vi "HFRR ADV v02.vi"() -> ()   [LabVIEW 2023] (continued)
            n1522 = Concatenate Strings("(" ("string"), w1758, ")  Deg C ," ("string")) -> (w1757:string)
            n1523 = Concatenate Strings("(" ("string"), w1754, " ) % RH," ("string")) -> (w1753:string)
            n1524 = Concatenate Strings("(" ("string"), w1750, ")  Deg C ," ("string")) -> (w1749:string)
            n1525 = Concatenate Strings("(" ("string"), w1747, ")  Microns," ("string")) -> (w1746:string)
            n1526 = local read "REMARKS"() -> (w1767:string)
            "REMARKS 2" <- w1767
            n1527 = Concatenate Strings(w1767, w1732, " Humidity before test= " ("Substring"), w1762, w1732, " Temperature before test = " ("Substring"), w1757, w1732, " Humidity after test= " ("Substring"), w1753, w1732, "Temperature after test = " ("Substring"), w1749, w1732, "MSD = " ("Substring"), w1746, w1732, "  AVP = " ("Substring"), w1733, w1732, "  HCF                     =( " ("Substring"), w1739, w1732, " WS1.4                  = " ("Substring"), w1735, w1732) -> (w1731:string)
            "data" <- w1731
            n1528 = call <vilib>:"Write Characters To File.vi"("append to file? (new file:F)"=FALSE, "character string"=w1731, "file path (dialog if empty)"=w1784) -> ()  [unwired: 2 in, 1 out]
            n1529 = Match Pattern(string=w1731, regular expression="!") -> (after substring=→"export":string)  [unwired: 1 in, 3 out]
          }
        }
        n1530 = local read "Temperature before test"() -> (w1700:dbl)
        n1531 = local read "Humidity before test"() -> (w1702:dbl)
        n1532 = local read "Temperature after test"() -> (w1716:dbl)
        n1533 = Add(x=231.864, y=w1700) -> (x+y=w1697:dbl)
        n1534 = Add(x=231.864, y=w1716) -> (x+y=w1713:dbl)
        n1535 = local read "Humidity after test"() -> (w1718:dbl)
        n1536 = Divide(x=1705.984, y=w1697) -> (x/y=w1698:dbl)
        n1537 = Divide(x=1705.984, y=w1713) -> (x/y=w1714:dbl)
        n1538 = Subtract(x=8.017352 ("y"), y=w1698) -> (x-y=w1727:dbl)
        n1539 = expression code="10**y"(w1727) -> (w1704:dbl)
        n1540 = Subtract(x=8.017352 ("y"), y=w1714) -> (x-y=w1721:dbl)
        n1541 = expression code="10**y"(w1721) -> (w1720:dbl)
        n1542 = Multiply(x=w1702, y=w1704) -> (x*y=w1703:dbl)
        n1543 = Multiply(x=w1718, y=w1720) -> (x*y=w1719:dbl)
        n1544 = Divide(x=w1703, y=750.0) -> (x/y=w1722:dbl)
        n1545 = Divide(x=w1719, y=750.0) -> (x/y=w1723:dbl)
        n1546 = Add(x=w1722, y=w1723) -> (x+y=w1724:dbl)
        n1547 = Divide(x=w1724, y=2.0) -> (x/y=w1726:dbl)
        n1548 = local write "AVP"(w1726) -> ()
        n1549 = local read "HCF"() -> (w1709:dbl)
        n1550 = Subtract(x=1.4, y=w1726) -> (x-y=w1707:dbl)
        n1551 = local read "MWSD"() -> (w1705:dbl)
        n1552 = Multiply(x=w1707, y=w1709) -> (x*y=w1708:dbl)
        n1553 = Add(x=w1708, y=w1705) -> (x+y=→"WS1.4":dbl)
      }
    }
    n1554 = case shown="True" "Prog Uno" {
      frame False {
      }
      frame True {
        n1555 = stacked-sequence {
          frame #0 {
            n1556 = Delete(path (use dialog)=path "C:/LAB-IQ-NXT/UNOCOMPILE.bat" ("working directory")) -> ()  [unwired: 4 in, 3 out]
          }
          frame #1 {
            n1557 = local read "Com Port 1"() -> (w1297:refnum<visa-resource-name>)
            n1558 = Concatenate Strings("cmd.exe /c \"mode " ("command line"), w1297, ":1200,n,8,1\"\n" ("command line")) -> (w1302:string)
            n1559 = Concatenate Strings(w1302, "CD\\\nCD WinDucom\navrdude -C avrdude.conf -v -patmega328p -carduino -P" ("command line"), w1297, " -b115200 -D -Uflash:w:UNO_V20.hex:i\n" ("command line"), "\r") -> (w1304:string)
            "STR" <- w1304
            n1560 = call <vilib>:"Write Characters To File.vi"("append to file? (new file:F)"=FALSE, "character string"=w1304, "file path (dialog if empty)"=path "C:/LAB-IQ-NXT/UNOCOMPILE.bat" ("working directory")) -> ()  [unwired: 2 in, 1 out]
          }
          frame #2 {
            n1561 = case shown="True" "Case Constant\n(See Context Help) 10" {
              frame False {
              }
              frame True {
                w1310 = "cmd.exe  /c \"C:\\LAB-IQ-NXT\\UNOCOMPILE.bat\"" ("string")
                n1562 = call <vilib>:"System Exec.vi"("expected output size  (4096)"=u32 65535, "run minimized? (F)"=FALSE, "wait until completion? (T)"=TRUE ("run minimized? (F)"), "working directory"=path "C:/LAB-IQ-NXT", "standard input"=w1310, "command line"=w1310) -> ("error out"=w1309:errorcluster, "standard output"=→"String 42":string)  [unwired: 2 in, 2 out]
                "error out 3" <- w1309
                n1563 = flat-sequence {
                  tunnel: w1309 -> [_]
                  frame #0 {
                  }
                }
              }
            }
            n1564 = local write "Prog Uno"(FALSE ("run minimized? (F)")) -> ()
          }
        }
      }
    }
    n1565 = case shown="True" "Prog Due" {
      frame False {
      }
      frame True {
        n1566 = stacked-sequence {
          frame #0 {
            n1567 = Delete(path (use dialog)=path "C:/LAB-IQ-NXT/DUECOMPILE.bat" ("working directory")) -> ()  [unwired: 4 in, 3 out]
          }
          frame #1 {
            n1568 = case shown="True" "Case Constant\n(See Context Help) 11" {
              frame False {
              }
              frame True {
                n1569 = local read "visa due"() -> (w1278:string)
                n1570 = Concatenate Strings("cmd.exe /c \"mode " ("command line"), w1278, ":1200,n,8,1\"\n" ("command line")) -> (w1283:string)
                n1571 = Concatenate Strings(w1283, "CD\\\nCD WinDucom\nTIMEOUT 1\n bossac.exe -i -d --port=" ("command line"), w1278, " -U false -e -w -v -b DUE.bin -R\n" ("command line"), "\r") -> (w1285:string)
                "concatenated string 2" <- w1285
                n1572 = call <vilib>:"Write Characters To File.vi"("append to file? (new file:F)"=FALSE, "character string"=w1285, "file path (dialog if empty)"=path "C:/LAB-IQ-NXT/DUECOMPILE.bat" ("working directory")) -> ()  [unwired: 2 in, 1 out]
              }
            }
          }
          frame #2 {
            # "C:\\LAB-IQ-NXT\\DUECOMPILE.bat"
            n1573 = case shown="True" "Case Constant\n(See Context Help) 12" {
              frame False {
              }
              frame True {
                w1291 = "cmd.exe  /c \"C:\\LAB-IQ-NXT\\DUECOMPILE.bat\"" ("string")
                n1574 = call <vilib>:"System Exec.vi"("expected output size  (4096)"=u32 65535, "run minimized? (F)"=FALSE, "wait until completion? (T)"=TRUE ("run minimized? (F)"), "working directory"=path "C:/LAB-IQ-NXT", "standard input"=w1291, "command line"=w1291) -> ("error out"=w1290:errorcluster, "standard output"=→"String 44":string)  [unwired: 2 in, 2 out]
                "error out 4" <- w1290
                n1575 = flat-sequence {
                  tunnel: w1290 -> [_]
                  frame #0 {
                  }
                }
              }
            }
            n1576 = local write "Prog Due"(FALSE ("Prog Due")) -> ()
          }
        }
      }
    }
    n1577 = flat-sequence {
      frame #0 {
        n1578 = local read "x = y?"() -> (w1320:bool)
        n1579 = And(x="EDIT", y=w1320) -> (x .and. y?=w1318:bool)
        n1580 = case shown="True" "SAVE" {
          frame False {
          }
          frame True {
            n1581 = stacked-sequence {
              seq-local: [w1521 _ _] -> [_ w1677 _]
              frame #0 {
                (unwired) i16 5 ("precision (6)")
                # "[CH1]    - FF\n[CH2]   - TEMPERATURE\n[CH3]    - Humidity\n[CH4]    - AIR TEMP\n[CH5]\\- Visa Uno\n[CH6] \\- Visa Due\n[CH7]  \\- file path\n[CH8]   - Displacement Gain\n[CHA]   - Stroke Gain\n[CHB]   - Stroke PID Gain\n[CHC]   -Language Selection\n[CHD]   -Power +\n[CHE]   -Power_\n[CHF]   -Heater\n[CHG]   -Humidity Wet\n[CHH]   -Humidity Dry\n[CHI]   -Integral Time"
                n1582 = local read "Com Port 1"() -> (w1512:refnum<visa-resource-name>)
                n1583 = local read "AIR TEMPERATURE :"() -> (w1508:dbl)
                n1584 = local read "DISPLACEMENT :"() -> (w1506:dbl)
                n1585 = local read "HUMIDITY:"() -> (w1507:dbl)
                n1586 = local read "Com Port 2"() -> (w1511:refnum<visa-resource-name>)
                n1587 = local read "TEMPERATURE :"() -> (w1509:dbl)
                n1588 = local read "Stroke PID Gains"() -> (w1572:T5)
                n1589 = local read "FRIC. FORCE :"() -> (w1510:dbl)
                n1590 = local read "STROKE GAIN :"() -> (w1505:dbl)
                n1591 = Unbundle By Name(w1572) -> ("Proportional Gain (Kc)"=w1571:dbl, "Integral Time (Ti, min)"=w1513:dbl)
                n1592 = local read "CH-HUMIDITY DRY"() -> (w1524:u16)
                n1593 = Path To String(path="File Path") -> (string=w1594:string)
                n1594 = local read "Language Selection"() -> (w1569:enum16{"English", "Russian"})
                n1595 = local read "CH-POWER +"() -> (w1536:u16)
                n1596 = local read "CH-HUMIDITY WET"() -> (w1527:u16)
                n1597 = Number To Fractional String(number=w1507, width (-)=i16 10 ("precision (6)"), precision (6)=i16 5) -> (F-format string=w1619:string)  [unwired: 1 in]
                n1598 = Concatenate Strings(w1594, "\\" ("string")) -> (w1593:string)
                n1599 = local read "CH-POWER -"() -> (w1533:u16)
                n1600 = Number To Fractional String(number=w1509, width (-)=i16 10 ("precision (6)"), precision (6)=i16 5) -> (F-format string=w1625:string)  [unwired: 1 in]
                n1601 = Number To Fractional String(number=w1508, width (-)=i16 10 ("precision (6)"), precision (6)=i16 5) -> (F-format string=w1613:string)  [unwired: 1 in]
                n1602 = Number To Fractional String(number=w1506, width (-)=i16 10 ("precision (6)"), precision (6)=i16 5) -> (F-format string=w1586:string)  [unwired: 1 in]
                n1603 = local read "CH-HEATER"() -> (w1530:u16)
                n1604 = Number To Fractional String(number=w1505, width (-)=i16 10 ("precision (6)"), precision (6)=i16 5) -> (F-format string=w1585:string)  [unwired: 1 in]
                n1605 = Number To Fractional String(number=w1510, width (-)=i16 10 ("precision (6)"), precision (6)=i16 5) -> (F-format string=w1626:string)  [unwired: 1 in]
                n1606 = Number To Fractional String(number=w1571, width (-)=i16 10 ("precision (6)"), precision (6)=i16 5) -> (F-format string=w1573:string)  [unwired: 1 in]
                n1607 = Number To Fractional String(number=w1569, width (-)=i16 10 ("precision (6)"), precision (6)=i16 5) -> (F-format string=w1565:string)  [unwired: 1 in]
                n1608 = Number To Fractional String(number=w1536, width (-)=i16 10 ("precision (6)"), precision (6)=i16 5) -> (F-format string=w1559:string)  [unwired: 1 in]
                n1609 = Number To Fractional String(number=w1533, width (-)=i16 10 ("precision (6)"), precision (6)=i16 5) -> (F-format string=w1556:string)  [unwired: 1 in]
                n1610 = Number To Fractional String(number=w1530, width (-)=i16 10 ("precision (6)"), precision (6)=i16 5) -> (F-format string=w1551:string)  [unwired: 1 in]
                n1611 = Number To Fractional String(number=w1527, width (-)=i16 10 ("precision (6)"), precision (6)=i16 5) -> (F-format string=w1548:string)  [unwired: 1 in]
                n1612 = Number To Fractional String(number=w1524, width (-)=i16 10 ("precision (6)"), precision (6)=i16 5) -> (F-format string=w1543:string)  [unwired: 1 in]
                n1613 = Concatenate Strings("[CH1]" ("string"), w1626, " - FF" ("string"), "\r") -> (w1624:string)
                n1614 = Concatenate Strings("[CH3]" ("string"), w1619, " - Humidity" ("string"), "\r") -> (w1616:string)
                n1615 = Concatenate Strings("[CH7]" ("string"), w1593, "- file path" ("string"), "\r") -> (w1596:string)
                n1616 = Number To Fractional String(number=w1513, width (-)=i16 10 ("precision (6)"), precision (6)=i16 5) -> (F-format string=w1517:string)  [unwired: 1 in]
                n1617 = Concatenate Strings("[CH6]" ("string"), w1511, "- Visa Due" ("string"), "\r") -> (w1597:string)
                n1618 = Concatenate Strings("[CH8]" ("string"), w1586, "- Displacement Gain" ("string"), "\r") -> (w1589:string)
                n1619 = Concatenate Strings("[CHA]" ("string"), w1585, "- Stroke Gain" ("string"), "\r") -> (w1579:string)
                n1620 = Concatenate Strings("[CH5]" ("string"), w1512, "- Visa Uno" ("string"), "\r") -> (w1602:string)
                n1621 = Concatenate Strings("[CH4]" ("string"), w1613, " - AIR TEMP" ("string"), "\r") -> (w1609:string)
                n1622 = Concatenate Strings("[CH2]" ("string"), w1625, " - TEMPERATURE" ("string"), "\r") -> (w1623:string)
                n1623 = Concatenate Strings("[CHC]" ("string"), w1565, "-Language Selection" ("string"), "\r") -> (w1562:string)
                n1624 = Concatenate Strings("[CHD]" ("string"), w1559, "-Power +" ("string"), "\r") -> (w1541:string)
                n1625 = Concatenate Strings("[CHE]" ("string"), w1556, "-Power_" ("string"), "\r") -> (w1540:string)
                n1626 = Concatenate Strings("[CHF]" ("string"), w1551, "-Heater" ("string"), "\r") -> (w1539:string)
                n1627 = Concatenate Strings("[CHB]" ("string"), w1573, "- Stroke PID Gain" ("string"), "\r") -> (w1570:string)
                n1628 = Concatenate Strings("[CHG]" ("string"), w1548, "-Humidity Wet" ("string"), "\r") -> (w1538:string)
                n1629 = Concatenate Strings("[CHH]" ("string"), w1543, "-Humidity Dry" ("string"), "\r") -> (w1537:string)
                n1630 = Concatenate Strings("[CHI]" ("string"), w1517, "-Integral Time " ("string"), "\r") -> (w1514:string)
                n1631 = Concatenate Strings(w1624, w1623, w1616, w1609, w1602, w1597, w1596, w1589, w1579, w1570, w1562, w1541, w1540, w1539, w1538, w1537, w1514) -> (w1521:string)
                "gain" <- w1521
              }
              frame #1 {
                n1632 = local read "AIR TEMP INTERCEPT:"() -> (w1638:dbl)
                n1633 = local read "TEMP INTERCEPT:"() -> (w1637:dbl)
                n1634 = local read "Com Port 3"() -> (w1647:refnum<visa-resource-name>)
                n1635 = local read "LvdtOff"() -> (w1640:dbl)
                n1636 = Number To Fractional String(number=w1637, width (-)=i16 10 ("precision (6)"), precision (6)=i16 5) -> (F-format string=w1665:string)  [unwired: 1 in]
                n1637 = Number To Fractional String(number=w1638, width (-)=i16 10 ("precision (6)"), precision (6)=i16 5) -> (F-format string=w1672:string)  [unwired: 1 in]
                n1638 = Number To Fractional String(number=w1640, width (-)=i16 10 ("precision (6)"), precision (6)=i16 5) -> (F-format string=w1644:string)  [unwired: 1 in]
                n1639 = Concatenate Strings("[CHK]" ("string"), w1665, "-TEMP INTERCEPT" ("string"), "\r") -> (w1661:string)
                n1640 = Concatenate Strings("[CHJ]" ("string"), w1672, "-AIR TEMP INTERCEPT" ("string"), "\r") -> (w1662:string)
                n1641 = Concatenate Strings("[SNO]" ("string"), "S.NO", "-" ("string"), "\r") -> (w1657:string)
                n1642 = Concatenate Strings("[CHL]" ("string"), w1647, "- Visa humid" ("string"), "\r") -> (w1650:string)
                n1643 = Concatenate Strings("[CHI]" ("string"), w1644, "-LVDT Position Offset" ("string"), "\r") -> (w1639:string)
                n1644 = Concatenate Strings(w1677, w1662, w1661, w1657, w1650, w1639) -> (w1676:string)
                n1645 = local read "Gain path"() -> (w1655:string)
                n1646 = Concatenate Strings(w1655, "\\calibrate std ED hfrr.dcf") -> ()  [unwired: 1 out]
                n1647 = String To Path(string="C:\\LAB-IQ-NXT\\calibrate WO 2464.dcf") -> (path=w1648:path)
                n1648 = call <vilib>:"Write Characters To File.vi"("append to file? (new file:F)"=FALSE, "character string"=w1676, "file path (dialog if empty)"=w1648) -> ()  [unwired: 2 in, 1 out]
              }
              frame #2 {
                n1649 = local write "Lan flag"(0.0 ("Lan flag")) -> ()
                n1650 = local write "Re-Initialise"(TRUE ("Re-Initialise")) -> ()
                n1651 = local write "conststatus"(0.0 ("rpm value : 2")) -> ()
                n1652 = local write "SAVE"(FALSE ("OK Button 14")) -> ()
              }
            }
          }
        }
        n1653 = case shown="False" w1318 {
          tunnel: [u8 2 ("Disabled") u8 0 ("Disabled")] -> w1317
          tunnel: [w1682 TRUE ("Visible")] -> w1316
          frame False {
            w1682 = FALSE ("Visible")
            n1654 = local write "EDIT 2"(w1682) -> ()
          }
          frame True {
          }
        }
        n1655 = property on="Tab Control" class="TabCtl (strict)"("Visible"=w1316) -> ()  [unwired: 2 in, 2 out]
        n1656 = property on="EDIT 2" class="Bool (strict)"("Visible"=w1316) -> ()  [unwired: 2 in, 2 out]
        n1657 = property on="TEMPERATURE :" class="DigNum (strict)"("Disabled"=w1317) -> ()  [unwired: 2 in, 2 out]
        n1658 = property on="SAVE" class="Bool (strict)"("Visible"=w1316) -> ()  [unwired: 2 in, 2 out]
        n1659 = property on="AIR TEMPERATURE :" class="DigNum (strict)"("Disabled"=w1317) -> ()  [unwired: 2 in, 2 out]
        n1660 = property on="SPEED OUT:" class="DigNum (strict)"("Disabled"=w1317) -> ()  [unwired: 2 in, 2 out]
        n1661 = property on="HUMIDITY:" class="DigNum (strict)"("Disabled"=w1317) -> ()  [unwired: 2 in, 2 out]
        n1662 = property on="FRIC. FORCE :" class="DigNum (strict)"("Disabled"=w1317) -> ()  [unwired: 2 in, 2 out]
        n1663 = property on="Tab Control 7" class="TabCtl (strict)"("Disabled"=w1317) -> ()  [unwired: 2 in, 2 out]
        n1664 = property on="Language Selection" class="Enum (strict)"("Visible"=w1316) -> ()  [unwired: 2 in, 2 out]
        n1665 = property on="File Path" class="Path"("Disabled"=w1317) -> ()  [unwired: 2 in, 2 out]
        n1666 = property on="TEMP INTERCEPT:" class="DigNum (strict)"("Disabled"=w1317) -> ()  [unwired: 2 in, 2 out]
        n1667 = property on="visa due" class="CmbBox"("Disabled"=w1317) -> ()  [unwired: 2 in, 2 out]
        n1668 = property on="AIR TEMP INTERCEPT:" class="DigNum (strict)"("Disabled"=w1317) -> ()  [unwired: 2 in, 2 out]
        n1669 = property on="CH-HUMIDITY DRY" class="DigNum (strict)"("Disabled"=w1317) -> ()  [unwired: 2 in, 2 out]
        n1670 = property on="CH-HUMIDITY WET" class="DigNum (strict)"("Disabled"=w1317) -> ()  [unwired: 2 in, 2 out]
        n1671 = property on="CH-POWER -" class="DigNum (strict)"("Disabled"=w1317) -> ()  [unwired: 2 in, 2 out]
        n1672 = property on="CH-HEATER" class="DigNum (strict)"("Disabled"=w1317) -> ()  [unwired: 2 in, 2 out]
        n1673 = property on="CH-POWER +" class="DigNum (strict)"("Disabled"=w1317) -> ()  [unwired: 2 in, 2 out]
        n1674 = property on="SrvM CP" class="Bool (strict)"("Disabled"=w1317) -> ()  [unwired: 2 in, 2 out]
        n1675 = property on="Stroke PID Gains" class="Clust (strict)"("Disabled"=w1317) -> ()  [unwired: 2 in, 2 out]
        n1676 = property on="STROKE GAIN :" class="DigNum (strict)"("Disabled"=w1317) -> ()  [unwired: 2 in, 2 out]
        n1677 = property on="LvdtOff" class="DigNum (strict)"("Disabled"=w1317) -> ()  [unwired: 2 in, 2 out]
        n1678 = property on="DISPLACEMENT :" class="DigNum (strict)"("Disabled"=w1317) -> ()  [unwired: 2 in, 2 out]
        n1679 = property on="Port 2 Error" class="Clust (strict)"("Visible"="EDIT") -> ()  [unwired: 2 in, 2 out]
        n1680 = property on="Port 1 Error" class="Clust (strict)"("Visible"="EDIT") -> ()  [unwired: 2 in, 2 out]
        n1681 = stacked-sequence {
          frame #0 {
            n1682 = local read "EDIT"() -> (w1368:bool)
            n1683 = case shown="False" w1368 {
              tunnel: [u8 2 ("Disabled") u8 0 ("Disabled")] -> _
              frame False {
                w1370 = FALSE
                n1684 = local write "Password"("") -> ()
                n1685 = property on="ENTER THE NEW PASSWORD" class="Str"("Visible"=w1370) -> ()  [unwired: 2 in, 2 out]
                n1686 = property on="ENTER CURRENT PASSWORD" class="Str"("Visible"=w1370) -> ()  [unwired: 2 in, 2 out]
                n1687 = property on="SrvM CP" class="Bool (strict)"("Visible"=w1370) -> ()  [unwired: 2 in, 2 out]
                n1688 = property on="Password" class="Str"("Visible"=w1370) -> ()  [unwired: 2 in, 2 out]
                n1689 = local write "x = y?"(w1370) -> ()
                n1690 = local write "SrvM CP"(w1370) -> ()
                n1691 = property on="message" class="Str"("Visible"=w1370) -> ()  [unwired: 2 in, 2 out]
              }
              frame True {
                w1373 = TRUE
                n1692 = property on="SrvM CP" class="Bool (strict)"("Visible"=w1373) -> ()  [unwired: 2 in, 2 out]
                n1693 = property on="Password" class="Str"("Visible"=w1373) -> ()  [unwired: 2 in, 2 out]
              }
            }
            "dipl pwd" <- "@143$\n" ("dipl pwd")
          }
          frame #1 {
            # "Gain password"
            n1694 = String To Byte Array(string="ENTER CURRENT PASSWORD") -> (unsigned byte array=w1378:u8[])
            n1695 = Search 1D Array(1D array=w1378, element=u8 10) -> (index of element=w1381:i32)  [unwired: 1 in]
            n1696 = Index Array(array=w1378, index=w1381) -> (element=w1377:u8)
            n1697 = Equal?(x=w1377, y=10) -> (x = y?=w1375:bool)
            n1698 = case shown="True" w1375 {
              frame False {
                n1699 = property on="ENTER THE NEW PASSWORD" class="Str"("Visible"=FALSE) -> ()  [unwired: 2 in, 2 out]
              }
              frame True {
                # "password"
                # "change password logic"
                n1700 = local read "dipl pwd"() -> (w1388:string)
                n1701 = local read "ENTER CURRENT PASSWORD"() -> (w1394:string)
                n1702 = String To Byte Array(string=w1394) -> (unsigned byte array=w1396:u8[])
                n1703 = Array Size(array=w1396) -> (size(s)=w1393:i32)
                n1704 = String To Byte Array(string=w1388) -> (unsigned byte array=w1389:u8[])
                n1705 = Array Size(array=w1389) -> (size(s)=w1391:i32)
                n1706 = for {
                  N: w1393 -> [_]
                  tunnel: w1396 -> [w1420]
                  tunnel: [w1418] -> w1397 mode=indexing
                  tunnel: w1393 -> [w1412]
                  i -> [w1413]
                  n1707 = Decrement(x=w1412) -> (x-1=w1410:i32)
                  n1708 = Index Array(array=w1420, index=w1413) -> (element=w1414:u8)
                  n1709 = Equal?(x=w1413, y=w1410) -> (x = y?=w1411:bool)
                  n1710 = Number To Decimal String(number=w1414) -> (decimal integer string=w1419:string)  [unwired: 1 in]
                  n1711 = Select(t="", s=w1411, f="\r") -> (s? t:f=w1416:string)
                  n1712 = Concatenate Strings(w1419, w1416) -> (w1418:string)
                }
                n1713 = for {
                  N: w1391 -> [_]
                  tunnel: w1389 -> [w1408]
                  tunnel: [w1406] -> w1390 mode=indexing
                  tunnel: w1391 -> [w1403]
                  i -> [w1404]
                  n1714 = Decrement(x=w1403) -> (x-1=w1402:i32)
                  n1715 = Index Array(array=w1408, index=w1404) -> (element=w1407:u8)
                  n1716 = Equal?(x=w1404, y=w1402) -> (x = y?=w1401:bool)
                  n1717 = Number To Decimal String(number=w1407) -> (decimal integer string=w1405:string)  [unwired: 1 in]
                  n1718 = Select(t="", s=w1401, f="\r") -> (s? t:f=w1398:string)
                  n1719 = Concatenate Strings(w1405, w1398) -> (w1406:string)
                }
                n1720 = local read "string"() -> (w1395:string)
                n1721 = Concatenate Strings(w1397) -> (w1385:string)
                n1722 = Concatenate Strings(w1390) -> (w1384:string)
                n1723 = Concatenate Strings(w1395) -> (w1392:string)
                n1724 = Equal?(x=w1385, y=w1384) -> (x = y?=w1383:bool)
                n1725 = Equal?(x=w1385, y=w1392) -> (x = y?=w1387:bool)
                n1726 = Or(x=w1387, y=w1383) -> (x .or. y?=w1386:bool)
                n1727 = case shown="True" w1386 {
                  frame False {
                  }
                  frame True {
                    n1728 = property on="ENTER THE NEW PASSWORD" class="Str"("Visible"=TRUE) -> ()  [unwired: 2 in, 2 out]
                  }
                }
              }
            }
          }
          frame #2 {
            n1729 = String To Byte Array(string="ENTER THE NEW PASSWORD") -> (unsigned byte array=w1423:u8[])
            n1730 = Search 1D Array(1D array=w1423, element=u8 10) -> (index of element=w1427:i32)  [unwired: 1 in]
            n1731 = Index Array(array=w1423, index=w1427) -> (element=w1425:u8)
            n1732 = Equal?(x=w1425, y=10) -> (x = y?=w1422:bool)
            n1733 = case shown="True" w1422 {
              frame False {
              }
              frame True {
                n1734 = local read "ENTER THE NEW PASSWORD"() -> (w1430:string)
                n1735 = String To Byte Array(string=w1430) -> (unsigned byte array=w1435:u8[])
                n1736 = Array Size(array=w1435) -> (size(s)=w1432:i32)
                n1737 = for {
                  N: w1432 -> [_]
                  tunnel: w1435 -> [w1448]
                  tunnel: [w1445] -> w1437 mode=indexing
                  tunnel: w1432 -> [w1440]
                  i -> [w1438]
                  n1738 = Index Array(array=w1448, index=w1438) -> (element=w1447:u8)
                  n1739 = Decrement(x=w1440) -> (x-1=w1441:i32)
                  n1740 = Equal?(x=w1438, y=w1441) -> (x = y?=w1442:bool)
                  n1741 = Number To Decimal String(number=w1447) -> (decimal integer string=w1446:string)  [unwired: 1 in]
                  n1742 = Select(t="", s=w1442, f="\r") -> (s? t:f=w1439:string)
                  n1743 = Concatenate Strings(w1446, w1439) -> (w1445:string)
                }
                n1744 = local write "SrvM CP"(FALSE) -> ()
                n1745 = local write "EDIT"(FALSE) -> ()
                n1746 = local read "file path"() -> (w1429:path)
                n1747 = Concatenate Strings(w1437) -> (w1431:string)
                n1748 = Delete(path (use dialog)=w1429) -> (deleted path=w1433:path)  [unwired: 4 in, 2 out]
                n1749 = call <vilib>:"Write Characters To File.vi"("append to file? (new file:F)"=FALSE, "character string"=w1431, "file path (dialog if empty)"=w1433) -> ()  [unwired: 2 in, 1 out]
              }
            }
          }
          frame #3 {
            n1750 = case shown="True" "SrvM CP" {
              frame False {
                w1451 = ""
                n1751 = property on="ENTER CURRENT PASSWORD" class="Str"("Visible"=FALSE) -> ()  [unwired: 2 in, 2 out]
                n1752 = local write "ENTER CURRENT PASSWORD"(w1451) -> ()
                n1753 = local write "ENTER THE NEW PASSWORD"(w1451) -> ()
              }
              frame True {
                n1754 = property on="ENTER THE NEW PASSWORD" class="Str"() -> ("Visible"=w1452:bool)  [unwired: 2 in, 2 out]
                n1755 = Not(x=w1452) -> (.not. x?=w1453:bool)
                n1756 = property on="ENTER CURRENT PASSWORD" class="Str"("Visible"=w1453) -> ()  [unwired: 2 in, 2 out]
              }
            }
          }
          frame #4 {
            n1757 = String To Byte Array(string="Password") -> (unsigned byte array=w1460:u8[])
            n1758 = Search 1D Array(1D array=w1460, element=u8 10) -> (index of element=w1458:i32)  [unwired: 1 in]
            n1759 = Index Array(array=w1460, index=w1458) -> (element=w1459:u8)
            n1760 = Equal?(x=w1459, y=10) -> (x = y?=w1455:bool)
            n1761 = case shown="True" w1455 {
              frame False {
              }
              frame True {
                # "password"
                # "password"
                n1762 = local read "Password"() -> (w1473:string)
                n1763 = String To Byte Array(string=w1473) -> (unsigned byte array=w1476:u8[])
                n1764 = Array Size(array=w1476) -> (size(s)=w1471:i32)
                n1765 = local read "file path"() -> (w1461:path)
                n1766 = for {
                  N: w1471 -> [_]
                  tunnel: w1476 -> [w1493]
                  tunnel: [w1491] -> w1477 mode=indexing
                  tunnel: w1471 -> [w1488]
                  i -> [w1489]
                  n1767 = Decrement(x=w1488) -> (x-1=w1487:i32)
                  n1768 = Index Array(array=w1493, index=w1489) -> (element=w1492:u8)
                  n1769 = Equal?(x=w1489, y=w1487) -> (x = y?=w1486:bool)
                  n1770 = Number To Decimal String(number=w1492) -> (decimal integer string=w1490:string)  [unwired: 1 in]
                  n1771 = Select(t="", s=w1486, f="\r") -> (s? t:f=w1483:string)
                  n1772 = Concatenate Strings(w1490, w1483) -> (w1491:string)
                }
                n1773 = String To Byte Array(string="@143$\n") -> (unsigned byte array=w1462:u8[])
                n1774 = Array Size(array=w1462) -> (size(s)=w1467:i32)
                n1775 = call <vilib>:"Read Characters From File.vi"("file path (dialog if empty)"=w1461) -> ("character string"=w1475:string)  [unwired: 5 in, 3 out]
                "string" <- w1475
                n1776 = for {
                  N: w1467 -> [_]
                  tunnel: w1462 -> [w1504]
                  tunnel: [w1502] -> w1465 mode=indexing
                  tunnel: w1467 -> [w1499]
                  i -> [w1500]
                  n1777 = Decrement(x=w1499) -> (x-1=w1498:i32)
                  n1778 = Index Array(array=w1504, index=w1500) -> (element=w1503:u8)
                  n1779 = Equal?(x=w1500, y=w1498) -> (x = y?=w1497:bool)
                  n1780 = Number To Decimal String(number=w1503) -> (decimal integer string=w1501:string)  [unwired: 1 in]
                  n1781 = Select(t="", s=w1497, f="\r") -> (s? t:f=w1494:string)
                  n1782 = Concatenate Strings(w1501, w1494) -> (w1502:string)
                }
                n1783 = Concatenate Strings(w1477) -> (w1469:string)
                n1784 = Concatenate Strings(w1475) -> (w1474:string)
                n1785 = Equal?(x=w1469, y=w1474) -> (x = y?=w1464:bool)
                n1786 = Concatenate Strings(w1465) -> (w1466:string)
                n1787 = Equal?(x=w1469, y=w1466) -> (x = y?=w1470:bool)
                n1788 = Or(x=w1464, y=w1470) -> (x .or. y?=w1463:bool)
                "x = y?" <- w1463
                n1789 = case shown="True" w1463 {
                  selector: w1463 -> [w1480 _]
                  tunnel: w1472 -> [_ _]
                  frame False {
                    n1790 = And(x=w1480, y=TRUE ("Visible")) -> (x .and. y?=w1481:bool)
                    n1791 = property on="message" class="Str"("Visible"=w1481) -> ()  [unwired: 2 in, 2 out]
                  }
                  frame True {
                    n1792 = property on="message" class="Str"("Visible"=FALSE) -> ()  [unwired: 2 in, 2 out]
                  }
                }
                n1793 = flat-sequence {
                  tunnel: [w1478] -> w1472
                  frame #0 {
                    w1478 = ""
                    n1794 = local write "Password"(w1478) -> ()
                  }
                }
              }
            }
          }
        }
        n1795 = case shown="True" "SrvM CP 2" {
          frame False {
          }
          frame True {
            n1796 = local read "FRIC. FORCE : 2"() -> (w1366:dbl)
            n1797 = local read "STROKE GAIN : 2"() -> (w1365:dbl)
            n1798 = local read "TEMPERATURE : 2"() -> (w1363:dbl)
            n1799 = local read "HUMIDITY: 2"() -> (w1361:dbl)
            n1800 = local read "DISPLACEMENT : 4"() -> (w1364:dbl)
            n1801 = local read "AIR TEMPERATURE : 2"() -> (w1362:dbl)
            n1802 = local read "TEMP INTERCEPT: 2"() -> (w1360:dbl)
            n1803 = local read "AIR TEMP INTERCEPT: 2"() -> (w1359:dbl)
            n1804 = local write "FRIC. FORCE :"(w1366) -> ()
            n1805 = local write "STROKE GAIN :"(w1365) -> ()
            n1806 = local write "TEMPERATURE :"(w1363) -> ()
            n1807 = local write "AIR TEMPERATURE :"(w1362) -> ()
            n1808 = local write "HUMIDITY:"(w1361) -> ()
            n1809 = local write "DISPLACEMENT :"(w1364) -> ()
            n1810 = local write "AIR TEMP INTERCEPT:"(w1360) -> ()
            n1811 = local write "TEMP INTERCEPT:"(w1359) -> ()
            n1812 = local write "SrvM CP 2"(FALSE ("SrvM CP 2")) -> ()
          }
        }
        n1813 = local read "STROKE GAIN : 2"() -> (w1335:dbl)
        n1814 = local read "FRIC. FORCE : 2"() -> (w1338:dbl)
        n1815 = local read "AIR TEMPERATURE : 2"() -> (w1326:dbl)
        n1816 = local read "DISPLACEMENT : 4"() -> (w1331:dbl)
        n1817 = local read "TEMPERATURE : 2"() -> (w1329:dbl)
        n1818 = local read "STROKE GAIN :"() -> (w1334:dbl)
        n1819 = local read "HUMIDITY: 2"() -> (w1322:dbl)
        n1820 = local read "FRIC. FORCE :"() -> (w1337:dbl)
        n1821 = local read "AIR TEMPERATURE :"() -> (w1325:dbl)
        n1822 = local read "DISPLACEMENT :"() -> (w1330:dbl)
        n1823 = local read "TEMPERATURE :"() -> (w1327:dbl)
        n1824 = local read "HUMIDITY:"() -> (w1321:dbl)
        n1825 = Subtract(x=w1322, y=w1321) -> (x-y=w1323:dbl)
        n1826 = Subtract(x=w1335, y=w1334) -> (x-y=w1333:dbl)
        n1827 = Subtract(x=w1338, y=w1337) -> (x-y=w1336:dbl)
        n1828 = Subtract(x=w1329, y=w1327) -> (x-y=w1328:dbl)
        n1829 = Subtract(x=w1331, y=w1330) -> (x-y=w1332:dbl)
        n1830 = Subtract(x=w1326, y=w1325) -> (x-y=w1324:dbl)
        n1831 = Divide(x=w1333, y=w1334) -> (x/y=w1353:dbl)
        n1832 = Divide(x=w1324, y=w1325) -> (x/y=w1348:dbl)
        n1833 = Divide(x=w1336, y=w1337) -> (x/y=w1356:dbl)
        n1834 = Divide(x=w1323, y=w1321) -> (x/y=w1345:dbl)
        n1835 = Divide(x=w1328, y=w1327) -> (x/y=w1349:dbl)
        n1836 = Divide(x=w1332, y=w1330) -> (x/y=w1352:dbl)
        n1837 = Multiply(x=w1353, y=100.0) -> (x*y=→"STROKE Calibration Error":dbl)
        n1838 = Multiply(x=w1348, y=100.0) -> (x*y=→"AIR TEMPERATURE  Calibration Error":dbl)
        n1839 = Multiply(x=w1356, y=100.0) -> (x*y=→"FRIC. FORCE Calibration Error":dbl)
        n1840 = Multiply(x=w1352, y=100.0) -> (x*y=→"DISPLACEMENT  Calibration Error":dbl)
        n1841 = Multiply(x=w1345, y=100.0) -> (x*y=→"HUMIDITY  Calibration Error":dbl)
        n1842 = Multiply(x=w1349, y=100.0) -> (x*y=→"TEMPERATURE  Calibration Error":dbl)
      }
    }
  }
  n1843 = while {
    tunnel: [w2809] -> _
    tunnel: [w2808] -> w42
    tunnel: w16 -> [_]
    i -> [w2809]
    stop <- w2808 stop-if-true
    n1844 = local read "Main Tab"() -> (w2792:T1)
    n1845 = local read "Main Tab"() -> (w2794:T1)
    n1846 = local read "EDIT"() -> (w2815:bool)
    n1847 = case shown="True" w2815 {
      tunnel: [FALSE TRUE] -> w2800
      frame False {
      }
      frame True {
      }
    }
    n1848 = case shown="\"About\"" w2792 {
      frame "Acquire" {
      }
      frame "Compare Files", Default {
      }
      frame "About" {
      }
    }
    n1849 = local read "Rate"() -> (w2814:dbl)
    n1850 = Divide(x=1.0, y=w2814) -> (x/y=w2810:dbl)
    "Time 2" <- w2810
    n1851 = property on="Time slide" class="Slide (strict)"("Scale.Range:Maximum"=2500.0) -> ()  [unwired: 2 in, 2 out]
    n1852 = local read "conststatus"() -> (w2796:dbl)
    n1853 = Equal?(x=w2794, y=T10."About" ("Main Tab")) -> (x = y?=w2806:bool)
    n1854 = property on="FF Calibration g" class="WFGraph (strict)"("Visible"=w2800) -> ()  [unwired: 2 in, 2 out]
    n1855 = property on="Lift" class="Bool (strict)"("Visible"=w2800) -> ()  [unwired: 2 in, 2 out]
    n1856 = property on="Threshold" class="DigNum (strict)"("Visible"=w2800) -> ()  [unwired: 2 in, 2 out]
    n1857 = property on="Time slide" class="Slide (strict)"("Visible"=w2800) -> ()  [unwired: 2 in, 2 out]
    n1858 = Select(t=u32 2500 ("milliseconds to wait"), s=w2806, f=u32 500 ("milliseconds to wait")) -> (s? t:f=w2804:u32)
    n1859 = Multiply(x=w2810, y=w2804) -> (x*y=w2812:dbl)
    n1860 = Wait (ms)(milliseconds to wait=u32 50) -> ()  [unwired: 1 out]
    n1861 = call "Elapsed Time2"("Time Target (s)"=w2812, "Auto Reset"=TRUE) -> ("Time has Elapsed"=w2801:bool)  [unwired: 10 in, 7 out]
    n1862 = Equal?(x=w2796, y=0.0) -> (x = y?=w2797:bool)
    n1863 = case shown="True" w2797 {
      frame False {
      }
      frame True {
        # "C:\\WinDucom\\calibrate WO 2391.dcf"
        n1864 = local write "Lan flag"(22) -> ()
        n1865 = local write "conststatus"(10.0 ("rpm value : 2")) -> ()
        n1866 = String To Path(string="C:\\LAB-IQ-NXT\\calibrate WO 2464.dcf") -> (path=w2821:path)
        n1867 = Open/Create/Replace File "Open File"(file path (use dialog)=w2821) -> (refnum out=w2819:refnum<file>)  [unwired: 5 in, 2 out]
        n1868 = for {
          N: 22 -> [_]
          tunnel: w2819 -> [w2830]
          i -> [w2824]
          (unwired) TRUE ("line mode (F)")
          n1869 = Read from Text File "Read File"(file (use dialog)=w2830) -> (text=w2829:string)  [unwired: 3 in, 3 out]
          n1870 = Match Pattern(string=w2829, regular expression="]") -> (after substring=w2827:string)  [unwired: 1 in, 3 out]
          n1871 = String Subset(string=w2829, offset (0)=5, length (rest)=10 ("length (rest)")) -> (substring=w2822:string)
          n1872 = Fract/Exp String To Number(string=w2822) -> (number=w2823:dbl)  [unwired: 3 in, 1 out]
          n1873 = Match Pattern(string=w2827, regular expression="-") -> (before substring=w2825:string)  [unwired: 1 in, 3 out]
          n1874 = case shown="0" w2824 {
            tunnel: w2823 -> [w2833 w2834 w2835 w2836 _ _ _ w2841 w2842 w2843 w2846 w2847 w2848 w2849 w2850 w2851 w2852 w2855 w2856 _ _ w2859 _]
            tunnel: w2825 -> [_ _ _ _ w2837 w2838 w2839 _ _ _ _ _ _ _ _ _ _ _ _ w2857 w2858 _ _]
            frame 0 {
              n1875 = local write "FRIC. FORCE :"(w2833) -> ()
            }
            frame 1 {
              n1876 = local write "TEMPERATURE :"(w2834) -> ()
            }
            frame 2 {
              n1877 = local write "HUMIDITY:"(w2835) -> ()
            }
            frame 3 {
              n1878 = local write "AIR TEMPERATURE :"(w2836) -> ()
            }
            frame 4 {
              n1879 = local write "Com Port 1"(w2837) -> ()
            }
            frame 5 {
              n1880 = local write "visa due"(w2838) -> ()
              n1881 = local write "Com Port 2"(w2838) -> ()
            }
            frame 6 {
              n1882 = String To Path(string=w2839) -> (path=w2840:path)
              n1883 = local write "File Path"(w2840) -> ()
              "String" <- w2839
            }
            frame 7 {
              n1884 = local write "DISPLACEMENT :"(w2841) -> ()
            }
            frame 8 {
              n1885 = local write "STROKE GAIN :"(w2842) -> ()
            }
            frame 9 {
              n1886 = local read "Stroke PID Gains"() -> (w2845:T5)
              n1887 = Bundle By Name(cluster=w2845, "Proportional Gain (Kc)"=w2843) -> (w2844:T5)
              n1888 = local write "Stroke PID Gains"(w2844) -> ()
            }
            frame 10 {
              n1889 = local write "Language Selection"(w2846) -> ()
            }
            frame 11 {
              n1890 = local write "CH-POWER +"(w2847) -> ()
            }
            frame 12 {
              n1891 = local write "CH-POWER -"(w2848) -> ()
            }
            frame 13 {
              n1892 = local write "CH-HEATER"(w2849) -> ()
            }
            frame 14 {
              n1893 = local write "CH-HUMIDITY WET"(w2850) -> ()
            }
            frame 15 {
              n1894 = local write "CH-HUMIDITY DRY"(w2851) -> ()
            }
            frame 16 {
              n1895 = local read "Stroke PID Gains"() -> (w2854:T5)
              n1896 = Bundle By Name(cluster=w2854, "Integral Time (Ti, min)"=w2852) -> (w2853:T5)
              n1897 = local write "Stroke PID Gains"(w2853) -> ()
            }
            frame 17 {
              n1898 = local write "AIR TEMP INTERCEPT:"(w2855) -> ()
            }
            frame 18 {
              n1899 = local write "TEMP INTERCEPT:"(w2856) -> ()
            }
            frame 19 {
              n1900 = local write "S.NO"(w2857) -> ()
            }
            frame 20 {
              n1901 = local write "Com Port 3"(w2858) -> ()
            }
            frame 21 {
              n1902 = local write "LvdtOff"(w2859) -> ()
            }
            frame 22, Default {
            }
          }
        }
      }
    }
    n1903 = case shown="True" w2801 {
      frame False {
        # "79.77669138"
        # "2.3554"
        n1904 = local read "FRIC. FORCE :"() -> (w2864:dbl)
        n1905 = local read "FF cal val"() -> (w2861:dbl[])
        n1906 = Multiply(x=w2864, y=79.77669138) -> (x*y=w2863:dbl)
        n1907 = Multiply(x=w2861, y=w2863) -> (x*y=→"FF Calibration g":dbl[])
        "Err Count" <- 0 ("y")
      }
      frame True {
        n1908 = stacked-sequence {
          frame #0 {
            n1909 = stacked-sequence {
              frame #0 {
                "Lift" <- TRUE ("Lift")
              }
            }
          }
          frame #1 {
            w2876 = 2500 ("y")
            n1910 = local read "FF1"() -> (w2871:dbl[])
            n1911 = local read "Ch1"() -> (w2867:dbl[])
            "Waveform Chart 2" <- w2867
            n1912 = Array Size(array=w2871) -> (size(s)=w2870:i32)
            n1913 = Insert Into Array(array=w2871, index=w2870, new element=w2867) -> (w2873:dbl[])
            n1914 = call-poly <vilib>:"Mean.vi"("X"=w2867) -> ("mean"=→"Raw Mean":dbl)  [unwired: 1 out]
            n1915 = local read "RUN"() -> (w2868:bool)
            n1916 = Array Size(array=w2873) -> (size(s)=w2877:i32)
            n1917 = case shown="False" w2868 {
              frame False {
                n1918 = local write "Frequency"(0.0 ("Frequency")) -> ()
              }
              frame True {
              }
            }
            n1919 = Subtract(x=w2877, y=w2876) -> (x-y=w2875:i32)
            n1920 = Greater?(x=w2877, y=w2876) -> (0:w2878:bool)
            n1921 = case shown="True" w2878 {
              tunnel: w2875 -> [_ w2882]
              tunnel: [w2880 w2884] -> w2869
              tunnel: w2873 -> [w2880 w2883]
              frame False {
              }
              frame True {
                n1922 = Delete From Array(array=w2883, length=w2882, index=0) -> (array with subset deleted=w2884:dbl[])  [unwired: 1 out]
                "Numeric" <- w2882
              }
            }
            "FF1" <- w2869
            "PID Ref" <- TRUE ("PID Ref")
          }
          frame #2 {
          }
          frame #3 {
            w2885 = 0.0 ("lower limit")
            w2917 = 0.0 ("lower limit")
            # "CONVERT TO N"
            # "DATA PROCESSING"
            # "115 mV/N"
            n1923 = local read "Fric Val"() -> (w2978:dbl[])
            n1924 = local read "FRIC. FORCE :"() -> (w2968:dbl)
            n1925 = local read "Air temp"() -> (w2969:dbl[])
            n1926 = local read "temp buf"() -> (w2972:dbl[])
            n1927 = call-poly <vilib>:"Mean.vi"("X"=w2969) -> ("mean"=w2909:dbl)  [unwired: 1 out]
            "Raw air temp" <- w2909
            n1928 = local read "humid"() -> (w2919:string)
            n1929 = Multiply(x=w2978, y=1.0) -> (x*y=w2979:dbl[])
            n1930 = Multiply(x=w2968, y=79.77669138) -> (x*y=w2966:dbl)
            n1931 = call-poly <vilib>:"Mean.vi"("X"=w2972) -> ("mean"=w2911:dbl)  [unwired: 1 out]
            "Raw specimen temp" <- w2911
            n1932 = case shown="0, Default" "Calibrating" {
              tunnel: w2911 -> [w3001 _]
              tunnel: [w3001 w3002] -> w2910
              tunnel: w2909 -> [_ w3002]
              frame 0, Default {
              }
              frame 1 {
              }
            }
            n1933 = local read "HUMIDITY:"() -> (w2982:dbl)
            n1934 = Multiply(x=w2979, y=w2966) -> (x*y=w2976:dbl[])
            n1935 = Add(x=w2909, y="Offset Air Temp") -> (x+y=w2904:dbl)
            n1936 = local read "AIR TEMPERATURE :"() -> (w2953:dbl)
            n1937 = Fract/Exp String To Number(string=w2919) -> (number=w2918:dbl)  [unwired: 3 in, 1 out]
            n1938 = local read "TEMPERATURE :"() -> (w2952:dbl)
            n1939 = call-poly <vilib>:"Mean.vi"("X"=w2976) -> ("mean"=w2977:dbl)  [unwired: 1 out]
            n1940 = Multiply(x=w2918, y=w2982) -> (x*y=w2974:dbl)
            n1941 = Subtract(x=w2976, y=w2977) -> (x-y=w2915:dbl[])
            n1942 = case shown="True" "Boolean 4" {
              tunnel: w2910 -> [_ w3008]
              tunnel: "Standard Temp. ( °c )" -> [_ w3007]
              frame False {
              }
              frame True {
                n1943 = local read "Captured Values"() -> (w3005:dbl[][])
                n1944 = local write "Boolean 4"(FALSE ("Boolean 4")) -> ()
                n1945 = Build Array(w3007, w3008) -> (w3006:dbl[])
                n1946 = Build Array (concatenate)(w3005, w3006) -> (w3003:dbl[][])
                n1947 = local write "Captured Values"(w3003) -> ()
              }
            }
            n1948 = local read "AIR TEMP INTERCEPT:"() -> (w2949:dbl)
            n1949 = Multiply(x=w2904, y=w2953) -> (x*y=w2906:dbl)
            n1950 = Absolute Value(x=w2915) -> (abs(x)=w2983:dbl[])
            n1951 = Multiply(x=w2911, y=w2952) -> (x*y=w2905:dbl)
            n1952 = In Range and Coerce(upper limit=100.0, x=w2974, lower limit=w2917) -> (coerced(x)=w2921:dbl)  [unwired: 1 out]
            n1953 = local read "TEMP INTERCEPT:"() -> (w2916:dbl)
            n1954 = local read "Humid Last buf"() -> (w2944:dbl[])
            n1955 = call-poly <vilib>:"RMS.vi"("X"=w2915) -> ("rms value"=w2914:dbl)  [unwired: 1 out]
            n1956 = call-poly <vilib>:"Mean.vi"("X"=w2983) -> ()  [unwired: 2 out]
            n1957 = local read "RUN"() -> (w2965:bool)
            n1958 = Add(x=w2906, y=w2949) -> (x+y=w2951:dbl)
            n1959 = Add(x=w2905, y=w2916) -> (x+y=w2950:dbl)
            n1960 = local read "FRICVALZ"() -> (w2989:dbl)
            n1961 = Replace Array Subset(array=w2944, new element=w2921, index=0) -> (w2940:dbl[])
            n1962 = call <vilib>:"Mean PtByPt.vi"("x"=w2950, "sample length"=10) -> ("mean"=w2970:dbl)  [unwired: 2 in, 1 out]
            "TEMP 2" <- w2970
            n1963 = Select(t=0.01 ("FF fil1"), s=w2965, f=0.1 ("FF fil1")) -> (s? t:f=w2961:dbl)
            n1964 = case shown="True" "FRICVALZ 2" {
              tunnel: w2914 -> [_ w3025]
              frame False {
              }
              frame True {
                n1965 = local write "FRICVALZ 2"(FALSE ("FRICVALZ")) -> ()
                "FRICVALZ" <- w3025
              }
            }
            n1966 = Subtract(x=w2914, y=w2989) -> (x-y=w2980:dbl)
            n1967 = local read "AIR TEMP"() -> (w2958:dbl)
            n1968 = Multiply(x=w2951, y=w2961) -> (x*y=w2962:dbl)
            n1969 = Subtract(x=w2921, y=w2917) -> (x-y=w2920:dbl)
            "Humidity ( Rh )" <- w2920
            n1970 = Rotate 1D Array(1:w2940, 2:1 ("n")) -> (0:w2941:dbl[])
            n1971 = Index Array(array=w2940, index #1=0 ("index"), index #2=3 ("index")) -> (element #1=w2929:dbl, element #2=w2928:dbl)
            n1972 = case shown="True" "Boolean 5" {
              frame False {
              }
              frame True {
                n1973 = local write "Captured Values"(dbl[][] [] ("Captured Values")) -> ()
                n1974 = local write "Boolean 5"(FALSE) -> ()
                n1975 = local write "Best Fit"(dbl[] [] ("Best Fit")) -> ()
              }
            }
            n1976 = local read "FF 2"() -> (w2991:dbl)
            n1977 = Subtract(x=1.0 ("y"), y=w2961) -> (x-y=w2959:dbl)
            n1978 = Divide(x=w2929, y=w2928) -> (x/y=w2936:dbl)
            n1979 = Multiply(x=w2959, y=w2958) -> (x*y=w2957:dbl)
            n1980 = Multiply(x=w2980, y=0.1 ("FF fil1")) -> (x*y=w2995:dbl)
            n1981 = local write "TEMP"(w2970) -> ()
            n1982 = Multiply(x=0.9 ("FF fil2"), y=w2991) -> (x*y=w2994:dbl)
            n1983 = local write "Humid Last buf"(w2941) -> ()
            n1984 = Add(x=w2962, y=w2957) -> (x+y=w2955:dbl)
            n1985 = local read "offfset corr"() -> (w2932:bool)
            n1986 = local read "ecr buf"() -> (w2902:dbl[])
            n1987 = Subtract(x=1.0, y=w2936) -> (x-y=w2935:dbl)
            n1988 = Add(x=w2995, y=w2994) -> (x+y=w2988:dbl)
            "FF 2" <- w2988
            n1989 = local read "NORMAL LOAD"() -> (w2975:dbl)
            n1990 = Not A Number/Path/Refnum?(number/path/refnum=w2955) -> (NaN/Path/Refnum?=w2956:bool)
            n1991 = Absolute Value(x=w2935) -> (abs(x)=w2934:dbl)
            n1992 = Not(x=w2932) -> (.not. x?=w2930:bool)
            n1993 = Select(t=0.0, s=w2956, f=w2955) -> (s? t:f=w2887:dbl)
            "AIR TEMP" <- w2887
            n1994 = Greater Or Equal?(x=w2934, y=0.05) -> (x >= y?=w2923:bool)
            n1995 = call-poly <vilib>:"Mean.vi"("X"=w2902) -> ("mean"=w2899:dbl)  [unwired: 1 out]
            n1996 = And(x=w2923, y=w2930) -> (x .and. y?=w2931:bool)
            n1997 = Not A Number/Path/Refnum?(number/path/refnum=w2920) -> (NaN/Path/Refnum?=w2981:bool)
            n1998 = case shown="True" w2981 {
              frame False {
              }
              frame True {
                n1999 = local write "Humidity ( Rh )"(0.0 ("Humidity 3")) -> ()
              }
            }
            n2000 = case shown="True" w2931 {
              tunnel: w2929 -> [_ w3019]
              tunnel: w2928 -> [_ w3018]
              frame False {
                w3013 = 5.0 ("y")
                n2001 = local read "cnter"() -> (w3015:dbl)
                n2002 = Increment(x=w3015) -> (x+1=w3012:dbl)
                n2003 = Greater Or Equal?(x=w3012, y=w3013) -> (x >= y?=w3014:bool)
                n2004 = Select(t=w3013, s=w3014, f=w3012) -> (s? t:f=w3011:dbl)
                n2005 = local write "cnter"(w3011) -> ()
              }
              frame True {
                n2006 = Subtract(x=w3019, y=w3018) -> (x-y=→"offset":dbl)
                "offfset corr" <- TRUE ("offfset corr")
                "cnter" <- 0.0 ("cnter")
              }
            }
            n2007 = Multiply(x=w2899, y="ECR_Gain") -> (x*y=w2898:dbl)
            n2008 = local read "TEMP"() -> (w2987:dbl)
            n2009 = local read "ecr"() -> (w2893:dbl)
            n2010 = Divide(x=w2988, y=w2975) -> (x/y=w2945:dbl)
            n2011 = local read "offfset corr"() -> (w2925:bool)
            n2012 = Multiply(x=w2898, y=0.2) -> (x*y=w2891:dbl)
            n2013 = Multiply(x=0.8, y=w2893) -> (x*y=w2892:dbl)
            n2014 = call "Elapsed Time11"("Time Target (s)"=1.0) -> ("Time has Elapsed"=w2889:bool)  [unwired: 11 in, 7 out]
            n2015 = local read "cnter"() -> (w2927:dbl)
            n2016 = Not A Number/Path/Refnum?(number/path/refnum=w2987) -> (NaN/Path/Refnum?=w2986:bool)
            n2017 = Not A Number/Path/Refnum?(number/path/refnum=w2988) -> (NaN/Path/Refnum?=w2985:bool)
            n2018 = Not A Number/Path/Refnum?(number/path/refnum=w2945) -> (NaN/Path/Refnum?=w2947:bool)
            n2019 = Add(x=w2891, y=w2892) -> (x+y=w2890:dbl)
            n2020 = Select(t=0.0, s=w2947, f=w2945) -> (s? t:f=→"COF 2":dbl)
            n2021 = case shown="True" w2889 {
              tunnel: w2887 -> [_ w2997]
              frame False {
              }
              frame True {
                "AirT" <- w2997
              }
            }
            n2022 = Equal?(x=5.0 ("y"), y=w2927) -> (x = y?=w2926:bool)
            n2023 = Compound Arithmetic op=OR(w2986, w2985) -> (w2984:bool)
            n2024 = Not A Number/Path/Refnum?(number/path/refnum=w2890) -> (NaN/Path/Refnum?=w2900:bool)
            n2025 = Compound Arithmetic op=AND(w2923, w2926, w2925) -> (w2922:bool)
            n2026 = case shown="True" w2984 {
              frame False {
              }
              frame True {
                n2027 = local write "TEMP"(0.0 ("TEMP")) -> ()
                n2028 = local write "reinit"(TRUE ("reinit")) -> ()
                n2029 = local write "FF 2"(0.0 ("FF 2")) -> ()
              }
            }
            n2030 = Select(t=0.0, s=w2900, f=w2890) -> (s? t:f=w2897:dbl)
            n2031 = case shown="True" w2922 {
              frame False {
              }
              frame True {
                n2032 = local write "offfset corr"(FALSE ("offfset corr")) -> ()
                n2033 = local write "offset"(0.0 ("offset")) -> ()
              }
            }
            n2034 = In Range and Coerce(upper limit=100.0, x=w2897, lower limit=w2885) -> ()  [unwired: 2 out]
            "ecr" <- w2885
          }
          frame #4 {
            n2035 = case shown="True" "Boolean 6" {
              frame False {
              }
              frame True {
                n2036 = local read "Captured Values"() -> (w3037:dbl[][])
                n2037 = Index Array(array=w3037, index (col) #1=0 ("disabled index (col)"), index (col) #2=1 ("index (col)")) -> (element #1=w3035:dbl[], element #2=w3033:dbl[])  [unwired: 2 in]
                n2038 = local write "Boolean 6"(FALSE ("Boolean 6")) -> ()
                n2039 = call <vilib>:"Linear Fit.vi"("Y"=w3035, "X"=w3033) -> ("Best Linear Fit"=→"Best Fit":dbl[], "slope"=w3029:dbl, "intercept"=w3028:dbl)  [unwired: 9 in, 2 out]
                "Slope" <- w3029
                "Intercept" <- w3028
                n2040 = local read "Calibrating"() -> (w3030:u16)
                n2041 = case shown="1" w3030 {
                  tunnel: w3029 -> [w3039 w3041]
                  tunnel: w3028 -> [w3038 w3040]
                  frame 0, Default {
                    n2042 = local write "TEMPERATURE :"(w3039) -> ()
                    n2043 = local write "TEMP INTERCEPT:"(w3038) -> ()
                  }
                  frame 1 {
                    n2044 = local write "AIR TEMPERATURE :"(w3041) -> ()
                    n2045 = local write "AIR TEMP INTERCEPT:"(w3040) -> ()
                  }
                }
              }
            }
            n2046 = flat-sequence {
              frame #0 {
                n2047 = Wait (ms)(milliseconds to wait=u32 100) -> ()  [unwired: 1 out]
              }
              frame #1 {
                n2048 = local write "Lift"(FALSE ("Lift")) -> ()
              }
            }
          }
        }
      }
    }
    n2049 = local read "EXIT"() -> (w2808:bool)
    "Rate" <- 2500.0 ("No of Samples")
    "Humid Last buf" <- dbl[] [0.0, 0.0, 0.0, 0.0] ("Humid Last buf")
  }
  n2050 = VISA Close(VISA resource name=w12, error in (no error)=w11) -> (error out=w13:errorcluster)
  n2051 = call <vilib>:"Clear Errors.vi"("error in (no error)"=w13) -> ()  [unwired: 5 in, 2 out]
  n2052 = VISA Close(VISA resource name=w40, error in (no error)=w39) -> (error out=w37:errorcluster)
  n2053 = call <vilib>:"Clear Errors.vi"("error in (no error)"=w37) -> ()  [unwired: 5 in, 2 out]
  n2054 = Or(x=w27, y=w26) -> (x .or. y?=w28:bool)
  n2055 = while {
    tunnel: [w3103] -> w33
    shift-right: [w3083] -> _
    shift-left: "" -> [w3071]
    tunnel: [w3059] -> _
    i -> [w3059]
    stop <- w3103 stop-if-true
    w3085 = ";" ("string")
    n2056 = local read "start en"() -> (w3105:bool)
    n2057 = And(x="st enable", y=w3105) -> (x .and. y?=w3106:bool)
    n2058 = local read "ACQUIRE 3"() -> (w3048:bool)
    n2059 = local read "Elapsed time"() -> (w3067:dbl)
    n2060 = case shown="True" w3106 {
      tunnel: "st enable" -> [w3170 w3171]
      tunnel: [w3170 w3171] -> w3049
      frame False {
      }
      frame True {
        n2061 = local write "start en"(FALSE ("start en")) -> ()
      }
    }
    n2062 = Wait (ms)(milliseconds to wait=u32 80) -> ()  [unwired: 1 out]
    n2063 = local read "Stroke"() -> (w3058:dbl)
    n2064 = Greater?(x=w3067, y=0.1) -> (0:w3065:bool)
    n2065 = Or(x=w3049, y=w3048) -> (x .or. y?=w3050:bool)
    n2066 = case shown="True" "ACQUIRE 2" {
      frame False {
      }
      frame True {
        n2067 = call "Elapsed Time13"() -> ("Time has Elapsed"=w3113:bool)  [unwired: 12 in, 7 out]
        n2068 = case shown="True" w3113 {
          frame False {
          }
          frame True {
            n2069 = local write "ACQUIRE 2"(FALSE ("ACQUIRE 2")) -> ()
            n2070 = local write "ACQUIRE 3"(FALSE ("ACQUIRE 2")) -> ()
          }
        }
        n2071 = local write "ACQUIRE 3"(TRUE ("ACQUIRE 2")) -> ()
      }
    }
    n2072 = case shown="True" w3050 {
      tunnel: w3058 -> [_ w3193]
      tunnel: [w3173 _] -> w3102
      tunnel: w3065 -> [_ _]
      tunnel: w3048 -> [_ w3180]
      frame False {
        w3173 = TRUE ("PID Rst")
        n2073 = local read "stop cmd"() -> (w3174:bool)
        n2074 = case shown="True" w3174 {
          frame False {
          }
          frame True {
            n2075 = local write "stop cmd"(FALSE ("stop cmd")) -> ()
          }
        }
        n2076 = local write "PID Rst"(TRUE ("PID Rst")) -> ()
        "start en" <- w3173
      }
      frame True {
        w3200 = cluster{"output high":dbl, "output low":dbl} {"output high"=600.0, "output low"=-600.0} ("output range")
        n2077 = local read "STROKE GAIN :"() -> (w3185:dbl)
        n2078 = call "Elapsed Time6"("Reset"="PID Rst", "Auto Reset"=FALSE) -> ("Time has Elapsed"=w3194:bool)  [unwired: 10 in, 7 out]
        n2079 = Multiply(x="Set Strk", y=w3185) -> (x*y=w3178:dbl)
        n2080 = case shown="False" w3194 {
          tunnel: [w3205 w3206] -> w3197
          tunnel: "Set Strk" -> [w3205 _]
          tunnel: w3193 -> [_ w3206]
          frame False {
          }
          frame True {
          }
        }
        n2081 = Multiply(x=w3178, y=1.0) -> (x*y=w3177:dbl)
        n2082 = Select(t=T5 {"Proportional Gain (Kc)"=0.0, "Integral Time (Ti, min)"=0.02, "Derivative Time (Td, min)"=0.0} ("Stroke PID Gains"), s=w3180, f="Stroke PID Gains") -> (s? t:f=w3181:T5)
        n2083 = Not(x=w3194) -> (.not. x?=w3192:bool)
        n2084 = call-poly <vilib>:"PID.vi"("reinitialize? (F)"=w3192, "output range"=w3200, "PID gains"=w3181, "process variable"=w3197, "setpoint"="Set Strk") -> ("output"=w3191:dbl)  [unwired: 5 in, 1 out]
        "Slide 5" <- w3191
        n2085 = Select(t=w3191, s=w3194, f=0.0) -> (s? t:f=w3195:dbl)
        n2086 = flat-sequence {
          tunnel: w3195 -> [_]
          frame #0 {
            n2087 = local write "PID Rst"(FALSE ("PID Rst")) -> ()
          }
        }
        n2088 = Add(x=w3177, y=w3195) -> (x+y=w3190:dbl)
        n2089 = Unbundle(w3200) -> ("output high"=w3199:dbl, "output low"=w3198:dbl)
        n2090 = To Word Integer(number=w3190) -> (16bit integer=w3187:i16)
        n2091 = property on="Slide 5" class="Slide (strict)"("Scale.Range:Minimum"=w3198, "Scale.Range:Maximum"=w3199) -> ()  [unwired: 2 in, 2 out]
        n2092 = In Range and Coerce(upper limit=4095.0 ("f"), x=w3187, lower limit=100.0 ("f")) -> (coerced(x)=w3184:dbl)  [unwired: 1 out]
        "PID Out" <- w3184
        n2093 = Number To Decimal String(number=w3184) -> (decimal integer string=→"st gain":string)  [unwired: 1 in]
        "stop cmd" <- TRUE ("Auto Reset")
      }
    }
    n2094 = flat-sequence {
      frame #0 {
        n2095 = local read "CH-POWER +"() -> (w3117:u16)
        n2096 = local read "CH-POWER -"() -> (w3118:u16)
        n2097 = case shown="1" w3118 {
          tunnel: "PWR" -> [w3119 w3120 w3121 w3122 w3123 w3124 w3125 w3126]
          frame 0, Default {
            n2098 = local write "Do 0"(w3119) -> ()
          }
          frame 1 {
            n2099 = local write "Do 1"(w3120) -> ()
          }
          frame 2 {
            n2100 = local write "Do 2"(w3121) -> ()
          }
          frame 3 {
            n2101 = local write "Do 3"(w3122) -> ()
          }
          frame 4 {
            n2102 = local write "Do 4"(w3123) -> ()
          }
          frame 5 {
            n2103 = local write "Do 5"(w3124) -> ()
          }
          frame 6 {
            n2104 = local write "Do 6"(w3125) -> ()
          }
          frame 7 {
            n2105 = local write "Do 7"(w3126) -> ()
          }
        }
        n2106 = case shown="1" w3117 {
          tunnel: "PWR" -> [w3127 w3128 w3129 w3130 w3131 w3132 w3133 w3134]
          frame 0, Default {
            n2107 = local write "Do 0"(w3127) -> ()
          }
          frame 1 {
            n2108 = local write "Do 1"(w3128) -> ()
          }
          frame 2 {
            n2109 = local write "Do 2"(w3129) -> ()
          }
          frame 3 {
            n2110 = local write "Do 3"(w3130) -> ()
          }
          frame 4 {
            n2111 = local write "Do 4"(w3131) -> ()
          }
          frame 5 {
            n2112 = local write "Do 5"(w3132) -> ()
          }
          frame 6 {
            n2113 = local write "Do 6"(w3133) -> ()
          }
          frame 7 {
            n2114 = local write "Do 7"(w3134) -> ()
          }
        }
      }
    }
    n2115 = local read "RUN"() -> (w3056:bool)
    n2116 = Or(x=w3056, y="ACQUIRE 3") -> (x .or. y?=w3055:bool)
    n2117 = local read "Set Hz"() -> (w3073:dbl)
    n2118 = Select(t=w3073, s=w3055, f=0.0) -> (s? t:f=w3072:dbl)
    n2119 = local read "st gain"() -> (w3076:string)
    n2120 = local read "DO"() -> (w3077:string)
    n2121 = case shown="True" "Boolean 10" {
      frame False {
      }
      frame True {
        n2122 = local write "Tab Control 8"(enum32{"setup", "calibrate"}."calibrate" ("Tab Control 8")) -> ()
        n2123 = local write "Boolean 10"(FALSE ("Boolean 10")) -> ()
      }
    }
    n2124 = Number To Decimal String(number=w3072) -> (decimal integer string=w3075:string)  [unwired: 1 in]
    n2125 = case shown="True" "Boolean 11" {
      frame False {
      }
      frame True {
        n2126 = local write "Tab Control 8"(enum32{"setup", "calibrate"}."setup" ("Tab Control 8")) -> ()
